vi "TestClosePath.vi"(8 "error in (no error)":errorcluster) -> (0 "error out":errorcluster)   [LabVIEW 2019]
uses:
  PathCommands.ClosePath/PathCommands.ClosePath.lvclass
  PathCommands/Point.ctl
  <vilib>/addons/_JKI Toolkits/Caraya/classes/Assert/Assert Equal Value_Variant.vi
  <vilib>/addons/_JKI Toolkits/Caraya/classes/Test/Test.lvclass
  PathCommands/PathCommands.lvclass
  <vilib>/addons/_JKI Toolkits/Caraya/classes/Assert/Assert.lvclass
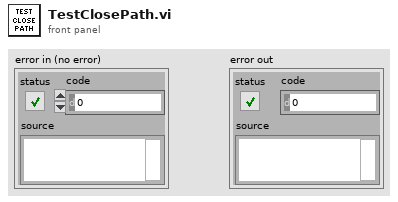
[diagram p1: front panel]
types:
  T1 = enum16{"None", "After", "Before", "Last", "First"}[]
  T2 = typedef "PathCommands.lvclass/Point.ctl" = cluster{"X":dbl, "Y":dbl}
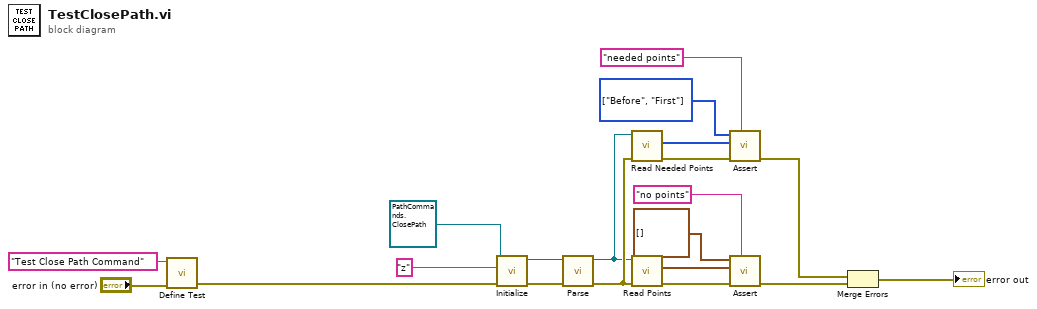
[diagram p0: block diagram]
diagram:
  w4 = T1 [enum."Before", enum."First"] items=["None", "After", "Before", "Last", "First"] ("Needed Points")
  n1 = call <vilib>:"Define Test.vi"("error in (no error)"="error in (no error)", "Label (VI Title)"="Test Close Path Command") -> ("error out"=w15:errorcluster)  [unwired: 8 in, 1 out]
  n2 = call-dynamic "Initialize.vi"("error in (no error)"=w15, "CommandText"="z", "PathCommands.ClosePath in"=refnum<class "PathCommands.ClosePath.lvclass"> refnum ("PathCommands.ClosePath.lvclass")) -> ("error out"=w18:errorcluster, "PathCommands.ClosePath out"=w19:refnum<class "PathCommands.ClosePath.lvclass">)  [unwired: 7 in]
  n3 = call-dynamic "Parse.vi"("error in (no error)"=w18, "PathCommands in"=w19) -> ("error out"=w8:errorcluster, "PathCommands out"=w7:refnum<class "PathCommands.ClosePath.lvclass">)  [unwired: 8 in]
  n4 = call-dynamic "Read Needed Points.vi"("error in (no error)"=w8, "PathCommands in"=w7) -> ("error out"=w6:errorcluster, "Needed Points"=w5:T1)  [unwired: 7 in, 1 out]
  n5 = call-dynamic "Read Points.vi"("error in (no error)"=w8, "PathCommands in"=w7) -> ("error out"=w12:errorcluster, "Points"=w13:T2[])  [unwired: 7 in, 1 out]
  n6 = call-poly <vilib>:"Assert.vi"("Label"="needed points", "error in (no error)"=w6, "Y"=w5, "X"=w4) -> ("error out"=w1:errorcluster)  [unwired: 6 in, 1 out]
  n7 = call-poly <vilib>:"Assert.vi"("Label"="no points", "error in (no error)"=w12, "Y"=w13, "X"=T2[] [] ("Points")) -> ("error out"=w11:errorcluster)  [unwired: 6 in, 1 out]
  n8 = Merge Errors(w1, w11) -> (→"error out":errorcluster)
